vi "JSON To Set.vi"(6 "LVClass Serializer":refnum<class "JSONtext LVClass Serializer.lvclass">, 8 "error in (no error)":errorcluster, 9 "Set Type":variant, 10 "Offset":i32, 11 "<JSON>":string) -> (0 "error out":errorcluster, 1 "Set":variant)   [LabVIEW 2020, in "JSONtext.lvlib" / "SetMap.lvlib"]
uses:
  <vilib>/JDP Science/JSONtext/support/Set Map/SetMap.lvlib
  <vilib>/JDP Science/JSONtext/LVClass Serializer/JSONtext LVClass Serializer.lvclass
  <vilib>/Utility/Data Type/NI_Data Type.lvlib
  <vilib>/JDP Science/JSONtext/JSONtext.lvlib
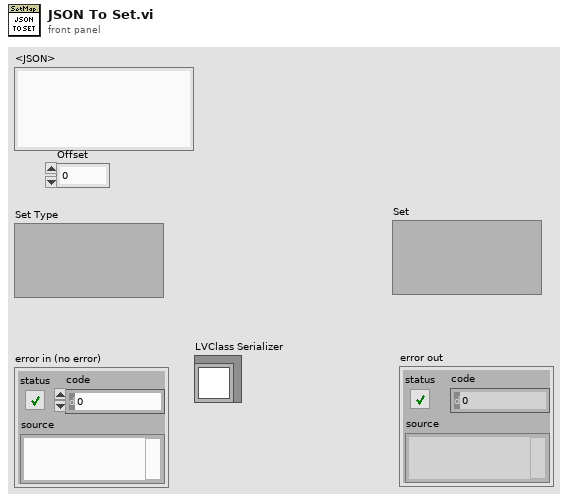
[diagram p1: front panel]
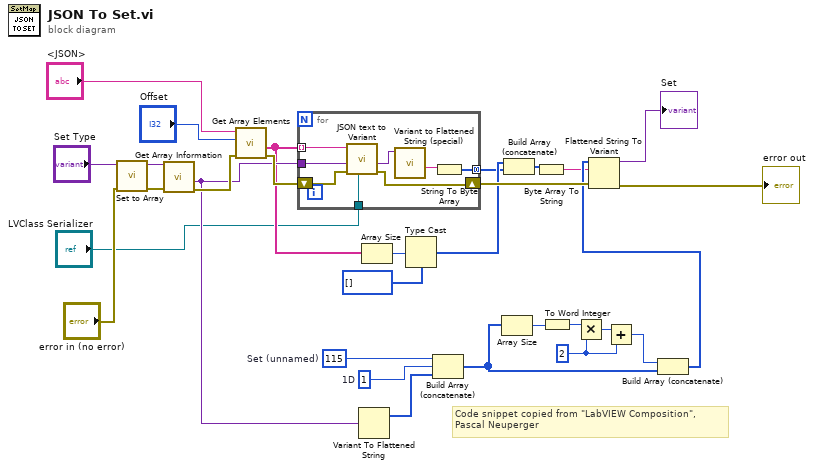
[diagram p0: block diagram]
diagram:
  w20 = i16 2 ("x")
  w14 = i16 1  # 1D
  w13 = i16 115  # Set (unnamed)
  # "Code snippet copied from \"LabVIEW Composition\",\nPascal Neuperger"
  n1 = call <vilib>:"Set to Array.vi"("error in"="error in (no error)", "Set"="Set Type") -> ("error out"=w25:errorcluster, "Array"=w3:variant)  [unwired: 8 in]
  n2 = call <vilib>:"Get Array Information.vi"("error in (no error)"=w25, "variant"=w3) -> ("error out"=w28:errorcluster, "array element data type"=w23:variant)  [unwired: 6 in, 2 out]
  n3 = call <vilib>:"Get Array Elements.vi"("error in (no error)"=w28, "Offset"="Offset", "JSON"="<JSON>") -> ("error out"=w29:errorcluster, "<JSON>"=w6:string[])  [unwired: 6 in, 1 out]
  n4 = for {
    tunnel: w6 -> [w38] mode=indexing
    tunnel: [w36] -> w10 mode=concatenating
    tunnel: w23 -> [w35]
    shift-right: [w33] -> w30
    shift-left: w29 -> [w34]
    tunnel: "LVClass Serializer" -> [w32]
    n5 = call <vilib>:"JSON text to Variant.vi"("LVClass Serializer"=w32, "error in (no error)"=w34, "Data Type"=w35, "JSON"=w38) -> ("error out"=w33:errorcluster, "Variant out"=w31:variant)  [unwired: 6 in]
    n6 = call <vilib>:"Variant to Flattened String (special).vi"("Variant"=w31) -> ("data"=w37:string)  [unwired: 9 in, 1 out]
    n7 = String To Byte Array(string=w37) -> (unsigned byte array=w36:u8[])
  }
  n8 = Variant To Flattened String(Variant=w23) -> (1:w12:i16[])  [unwired: 1 out]
  n9 = Array Size(array=w6) -> (size(s)=w5:i32)
  n10 = Type Cast(type=u8[] [], x=w5) -> (*(type *) &x=w11:u8[])
  n11 = Build Array (concatenate)(w13, w14, w12) -> (w16:i16[])
  n12 = Array Size(array=w16) -> (size(s)=w15:i32)
  n13 = Build Array (concatenate)(w11, w10) -> (w7:u8[])
  n14 = Byte Array To String(unsigned byte array=w7) -> (string=w9:string)
  n15 = To Word Integer(number=w15) -> (16bit integer=w17:i16)
  n16 = Multiply(x=w17, y=w20) -> (x*y=w18:i16)
  n17 = Add(x=w18, y=w20) -> (x+y=w19:i16)
  n18 = Build Array (concatenate)(w19, w16) -> (w21:i16[])
  n19 = Flattened String To Variant(4:w30, 6:w9, 7:w21) -> (0:→"error out":errorcluster, 3:→"Set":variant)
